vi "Populate Instrument List.vi"(4 "Seconds between samples":dbl=1.0 format="%_4f", 6 "Channels to scan (empty - don't use scanner option)":i32[](array[numeric]), 8 "error in (no error)":errorcluster, 11 "VISA Resourse Names":refnum<visa-resource-name>[](array[refnum])) -> (0 "error out":errorcluster, 3 "Instrument List":refnum<class "Instrument.lvclass">[](array[class]))   [LabVIEW 2015]
uses:
  Instrument.lvclass
  OO Devices/Device/Device type.ctl
  LakeShore/LakeShore340/LakeShore 340.lvclass
  LakeShore/LakeShore335/LakeShore 335.lvclass
  Keithley/Keithley 2400/Keithley2400.lvclass
  Oxford/ITC503/ITC 503.lvclass
  Oxford/IPS120/IPS120.lvclass
  LakeShore/LakeShore370/LakeShore370_device.lvclass
  HP/HP53181/HP53181.lvclass
  HP/HP53132/HP 53132.lvclass
  Neocera/Neocera LTC-21.lvclass
  Cryo-con/Cryo-Con-22C.lvclass
  SRS/sr850/SRS850.lvclass
  LR-700/LR-700.lvclass
  EG_G/5302/EGG5302.lvclass
  EG_G/EGG7260/EGG7260.lvclass
  EG_G/EGG7280/EGG7280.lvclass
  AH/AH2500.lvclass
  Keithley/Meter/KeithleyMeter.lvclass
  Keithley/Keithley 6220-6221/Keithley Source.lvclass
  Keithley/Electrometer/Keithley electrometer.lvclass
  HP/HP5385/HP5385.lvclass
  Cryomagnetics/Cryomagnetics Power Supply.lvclass
  Write VISA Resource.vi
  OO Devices/Device/Write Name.vi
  Instrument with scanner/Instrument with scanner.lvclass
panel:
  in  "Instrument":T1=enum."LkShr 340 chA&B"
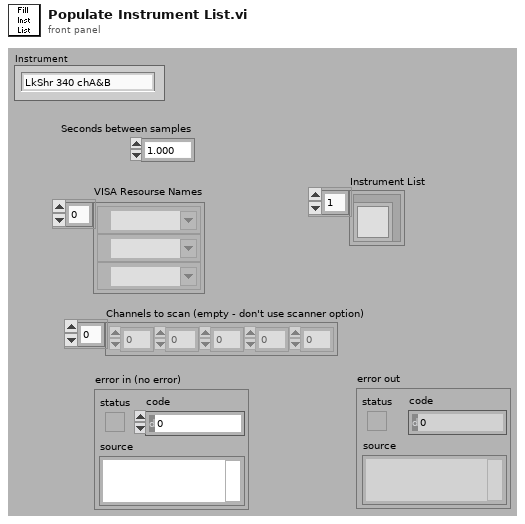
[diagram p1: front panel]
types:
  T1 = typedef "Device type.ctl" = enum16{"NONE", "Neocera 21", "LakeShore 335", "LakeShore 340", "LkShr 340 chA&B", "LakeShore 370", "SRS 850", "SRS 830", "LR 700", "EG&G 5302", "EG&G 7260", "EG&G 7280", "AH 2500", "Keithley meter", "Keithley electrometer", "Keithley 182", "HP 5385", "HP 53181", "HP 53132", "ITC503", "IPS120", "Oxford Mercury IPS", "Oxford PS", "Test", "DC Facility Magnet", "Cryomagnetics PS", "Keithley 2400", "Keithley current source", "Cryo-Con 22C", "HP87NN", "HP4395A"}
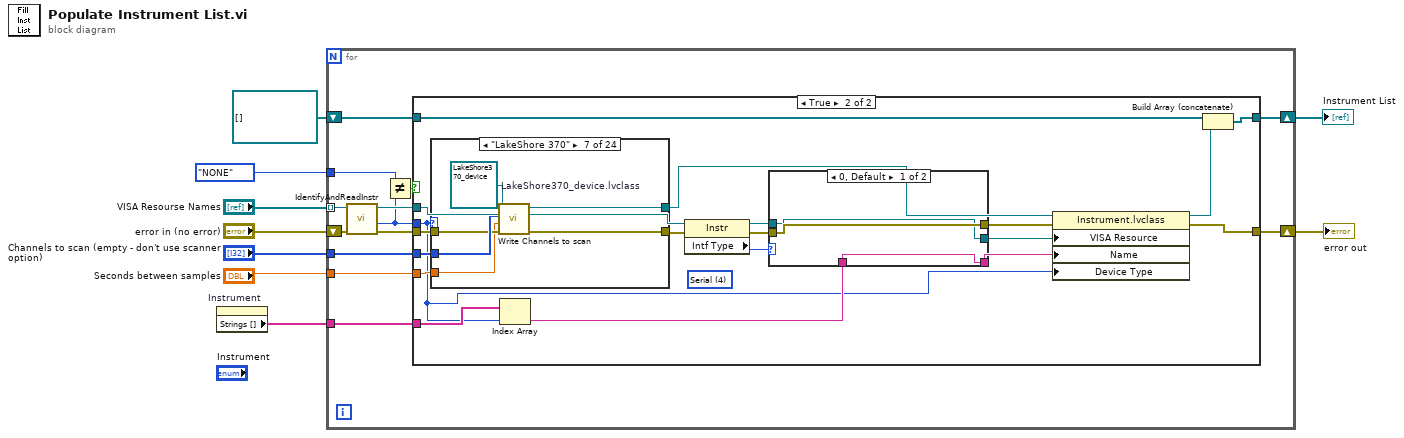
[diagram p0: block diagram]
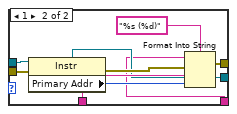
[diagram p3: hidden frame]
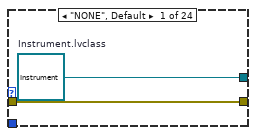
[diagram p4: hidden frame]
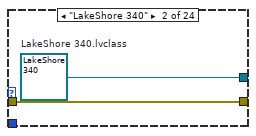
[diagram p5: hidden frame]
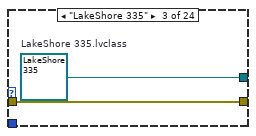
[diagram p6: hidden frame]
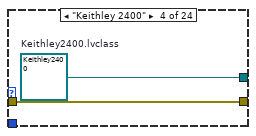
[diagram p7: hidden frame]
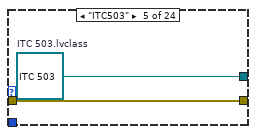
[diagram p8: hidden frame]
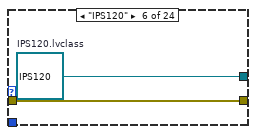
[diagram p9: hidden frame]
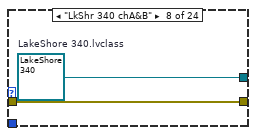
[diagram p10: hidden frame]
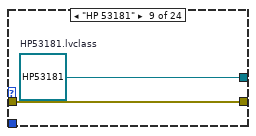
[diagram p11: hidden frame]
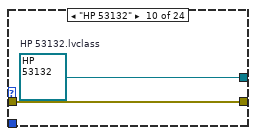
[diagram p12: hidden frame]
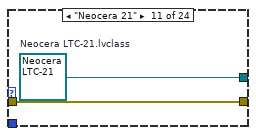
[diagram p13: hidden frame]
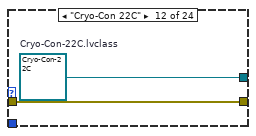
[diagram p14: hidden frame]
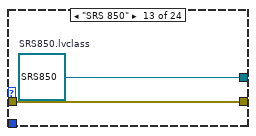
[diagram p15: hidden frame]
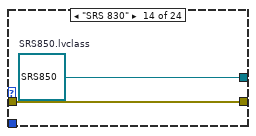
[diagram p16: hidden frame]
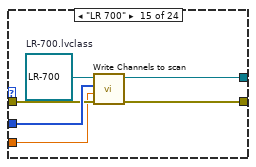
[diagram p17: hidden frame]
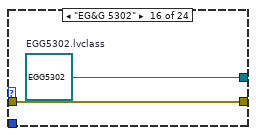
[diagram p18: hidden frame]
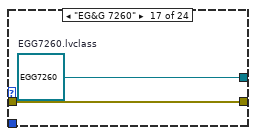
[diagram p19: hidden frame]
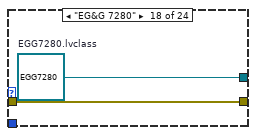
[diagram p20: hidden frame]
diagram:
  n1 = property on="Instrument" class="Enum (strict)"() -> ("Strings []"=w3:string[])  [unwired: 2 in, 2 out]
  n2 = for {
    tunnel: "VISA Resourse Names" -> [w20] mode=indexing
    shift-right: [w15] -> w7
    shift-left: "error in (no error)" -> [w22]
    tunnel: "Channels to scan (empty - don't use scanner option)" -> [w19]
    tunnel: "Seconds between samples" -> [w18]
    tunnel: w3 -> [w10]
    tunnel: Device_type."NONE" ("Instrument") -> [w13]
    shift-right: [w16] -> w6
    shift-left: refnum<class "Instrument.lvclass">[] [] -> [w11]
    n3 = call "IdentifyAndReadInstr.vi"("error in (no error)"=w22, "VISA Resource Name"=w20) -> ("error out"=w21:errorcluster, "Instrument"=w12:T1, "VISA Resource Name Out"=w17:refnum<visa-resource-name>)  [unwired: 7 out]
    n4 = Not Equal?(x=w13, y=w12) -> (x != y?=w14:bool)
    n5 = case shown="True" w14 {
      tunnel: w21 -> [w24 w43]
      tunnel: w19 -> [_ w41]
      tunnel: w18 -> [_ w40]
      tunnel: w17 -> [_ w28]
      tunnel: w12 -> [_ w30]
      tunnel: [w23 w39] -> w16
      tunnel: [w24 w31] -> w15
      tunnel: w11 -> [w23 w38]
      tunnel: w10 -> [_ w37]
      frame False {
      }
      frame True {
        (unwired) u16 4 items=["GPIB"=1, "VXI"=2, "GPIB-VXI"=3, "Serial"=4, "PXI"=5, "TCPIP"=6, "USB"=7, "FireWire"=9] ("Interface Information:Interface Type")
        n6 = case shown="\"LakeShore 370\"" w30 {
          tunnel: w43 -> [w57 w59 w61 w63 w64 w66 w71 w75 w77 w79 w81 w83 w85 w87 w90 w95 w97 w99 w101 w103 w105 w107 w109 w111]
          tunnel: [w57 w59 w61 w63 w64 w66 w70 w75 w77 w79 w81 w83 w85 w87 w89 w95 w97 w99 w101 w103 w105 w107 w109 w111] -> w27
          tunnel: [w56 w58 w60 w62 w65 w67 w73 w74 w76 w78 w80 w82 w84 w86 w92 w94 w96 w98 w100 w102 w104 w106 w108 w110] -> w42
          tunnel: w41 -> [_ _ _ _ _ _ w72 _ _ _ _ _ _ _ w91 _ _ _ _ _ _ _ _ _]
          tunnel: w40 -> [_ _ _ _ _ _ w69 _ _ _ _ _ _ _ w88 _ _ _ _ _ _ _ _ _]
          frame "NONE", Default {
            w56 = refnum<class "Instrument.lvclass"> refnum  # Instrument.lvclass
          }
          frame "LakeShore 340" {
            w58 = refnum<class "LakeShore 340.lvclass"> refnum  # LakeShore 340.lvclass
          }
          frame "LakeShore 335" {
            w60 = refnum<class "LakeShore 335.lvclass"> refnum  # LakeShore 335.lvclass
          }
          frame "Keithley 2400" {
            w62 = refnum<class "Keithley2400.lvclass"> refnum  # Keithley2400.lvclass
          }
          frame "ITC503" {
            w65 = refnum<class "ITC 503.lvclass"> refnum  # ITC 503.lvclass
          }
          frame "IPS120" {
            w67 = refnum<class "IPS120.lvclass"> refnum  # IPS120.lvclass
          }
          frame "LakeShore 370" {
            w68 = refnum<class "LakeShore370_device.lvclass"> refnum  # LakeShore370_device.lvclass
            n7 = call "Write Channels to scan.vi"("error in (no error)"=w71, "Seconds between samples"=w69, "Channels to scan (empty - don't use scanner option)"=w72, "Instrument with scanner.lvclass in"=w68) -> ("error out"=w70:errorcluster, "Instrument with scanner.lvclass out"=w73:refnum<class "LakeShore370_device.lvclass">)  [unwired: 6 out]
          }
          frame "LkShr 340 chA&B" {
            w74 = refnum<class "LakeShore 340.lvclass"> refnum  # LakeShore 340.lvclass
          }
          frame "HP 53181" {
            w76 = refnum<class "HP53181.lvclass"> refnum  # HP53181.lvclass
          }
          frame "HP 53132" {
            w78 = refnum<class "HP 53132.lvclass"> refnum  # HP 53132.lvclass
          }
          frame "Neocera 21" {
            w80 = refnum<class "Neocera LTC-21.lvclass"> refnum  # Neocera LTC-21.lvclass
          }
          frame "Cryo-Con 22C" {
            w82 = refnum<class "Cryo-Con-22C.lvclass"> refnum  # Cryo-Con-22C.lvclass
          }
          frame "SRS 850" {
            w84 = refnum<class "SRS850.lvclass"> refnum  # SRS850.lvclass
          }
          frame "SRS 830" {
            w86 = refnum<class "SRS850.lvclass"> refnum  # SRS850.lvclass
          }
          frame "LR 700" {
            w93 = refnum<class "LR-700.lvclass"> refnum  # LR-700.lvclass
            n8 = call "Write Channels to scan.vi"("error in (no error)"=w90, "Seconds between samples"=w88, "Channels to scan (empty - don't use scanner option)"=w91, "Instrument with scanner.lvclass in"=w93) -> ("error out"=w89:errorcluster, "Instrument with scanner.lvclass out"=w92:refnum<class "LR-700.lvclass">)  [unwired: 6 out]
          }
          frame "EG&G 5302" {
            w94 = refnum<class "EGG5302.lvclass"> refnum  # EGG5302.lvclass
          }
          frame "EG&G 7260" {
            w96 = refnum<class "EGG7260.lvclass"> refnum  # EGG7260.lvclass
          }
          frame "EG&G 7280" {
            w98 = refnum<class "EGG7280.lvclass"> refnum  # EGG7280.lvclass
          }
          frame "AH 2500" {
            w100 = refnum<class "AH2500.lvclass"> refnum  # AH2500.lvclass
          }
          frame "Keithley meter" {
            w102 = refnum<class "KeithleyMeter.lvclass"> refnum  # KeithleyMeter.lvclass
          }
          frame "Keithley current source" {
            w104 = refnum<class "Keithley Source.lvclass"> refnum  # Keithley Source.lvclass
          }
          frame "Keithley electrometer" {
            w106 = refnum<class "Keithley electrometer.lvclass"> refnum  # Keithley electrometer.lvclass
          }
          frame "HP 5385" {
            w108 = refnum<class "HP5385.lvclass"> refnum  # HP5385.lvclass
          }
          frame "Cryomagnetics PS" {
            w110 = refnum<class "Cryomagnetics Power Supply.lvclass"> refnum  # Cryomagnetics Power Supply.lvclass
          }
        }
        n9 = Index Array(array=w37, index=w30) -> (element=w36:string)
        n10 = property class="Instr"(reference=w28, error in=w27) -> (reference out=w29:refnum<visa-resource-name>, error out=w26:errorcluster, "Intf Type"=w25:u16)
        n11 = case shown="0, Default" w25 {
          tunnel: w36 -> [w44 w53]
          tunnel: [w45 w51] -> w35
          tunnel: [w44 w50] -> w34
          tunnel: [w46 w49] -> w32
          tunnel: w29 -> [w45 w48]
          tunnel: w26 -> [w46 w47]
          frame 0, Default {
          }
          frame 1 {
            n12 = property class="Instr"(reference=w48, error in=w47) -> (reference out=w51:refnum<visa-resource-name>, error out=w55:errorcluster, "Primary Addr"=w52:u16)
            n13 = Format Into String(format string="%s (%d)", error in=w55, w53, w52) -> (resulting string=w50:string, error out=w49:errorcluster)  [unwired: 1 in]
          }
        }
        n14 = property class="Instrument.lvclass"(reference=w42, error in=w32, "VISA Resource"=w35, "Name"=w34, "Device Type"=w30) -> (reference out=w33:refnum<class "Instrument.lvclass">, error out=w31:errorcluster)
        n15 = Build Array (concatenate)(w38, w33) -> (w39:refnum<class "Instrument.lvclass">[])
      }
    }
  }
  "error out" <- w7
  "Instrument List" <- w6
